vi "Finite_Geometric_Series.vi"() -> ()   [LabVIEW 2022 SP3]
panel:
  out "Percent Deviation":dbl format="%.5g"
  out "y∞":dbl format="%_5g"
  out "yN":dbl format="%_5g"
  in  "N":sgl format="%#_13g"
  in  "x":dbl
  # "Finite_Geometric_Series:"
  # "When x = 0.5, in order to get Percent Deviation below 0.1%, N must be 10.  This has a deviation of 0.09766, while a value of N = 9 returns a deviation of 0.19531"
  # "An infinite series of N terms is as follows:\nyN = x^0 + x^1 + x^2 + x^3 + …. x^N-1"
  # "After choosing a value of |x|<1 and N, see the \nPercent Difference between y∞ and yN"
  # "When N = ∞:  y∞ = 1/(1 - x)"
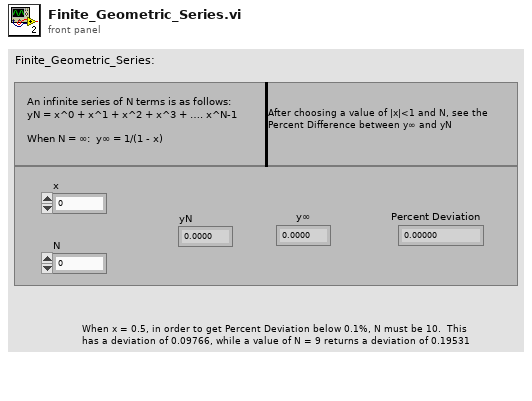
[diagram p1: front panel]
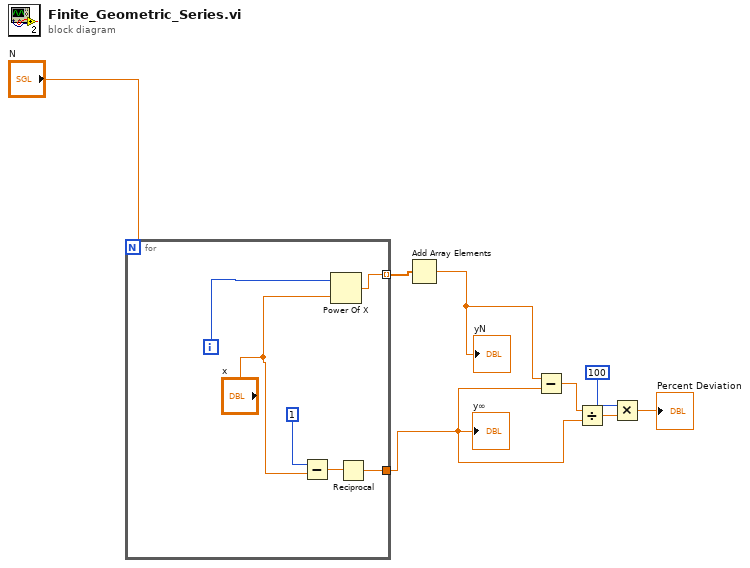
[diagram p0: block diagram]
diagram:
  n1 = for {
    N: "N" -> [_]
    tunnel: [w13] -> w7 mode=indexing
    tunnel: [w9] -> w4
    i -> [w14]
    n2 = Subtract(x=1, y="x") -> (x-y=w10:dbl)
    n3 = Power Of X(1:"x", 2:w14) -> (0:w13:dbl)
    n4 = Reciprocal(x=w10) -> (1/x=w9:dbl)
  }
  "y∞" <- w4
  n5 = Add Array Elements(numeric array=w7) -> (sum=w6:dbl)
  "yN" <- w6
  n6 = Subtract(x=w6, y=w4) -> (x-y=w5:dbl)
  n7 = Divide(x=w5, y=w4) -> (x/y=w3:dbl)
  n8 = Multiply(x=100, y=w3) -> (x*y=→"Percent Deviation":dbl)
